vi "__Cloud List Menu Download Handler.vi"(7 "FileManager Data":T1, 8 "error in (no error)":errorcluster) -> (0 "error out":errorcluster)   [LabVIEW 2011]
doc: "Handles the download operation on the cloud list."
uses:
  __File manager Data type.ctl
  vi.lib/National Instruments/LabVIEW Interface for Amazon S3/LV Interface for Amazon S3.lvlib
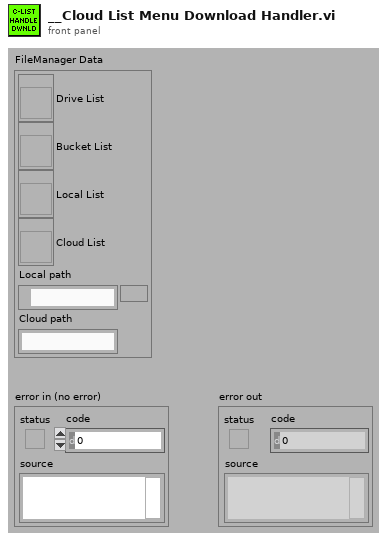
[diagram p1: front panel]
types:
  T1 = typedef "__File manager Data type.ctl" = cluster{"Drive List":refnum<vi>, "Bucket List":refnum<vi>, "Local List":refnum<vi>, "Cloud List":refnum<vi>, "Local path":path, "Cloud path":string}
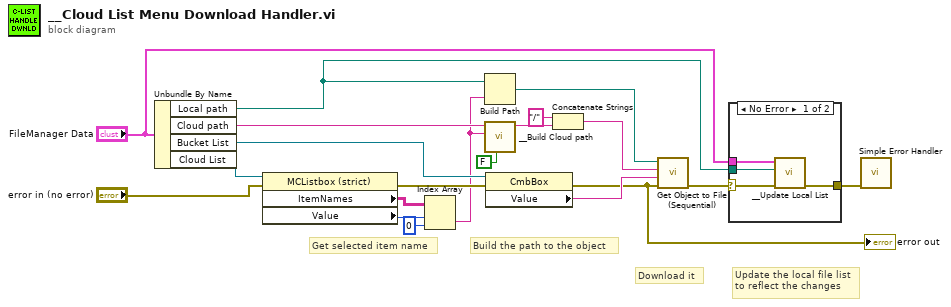
[diagram p0: block diagram]
diagram:
  # "Update the local file list\nto reflect the changes"
  # "Download it"
  # "Build the path to the object"
  # "Get selected item name"
  n1 = Unbundle By Name("FileManager Data") -> ("Local path"=w4:path, "Cloud path"=w13:string, "Bucket List"=w16:refnum<vi>, "Cloud List"=w20:refnum<vi>)
  n2 = property class="MCListbox (strict)"(reference=w20, error in="error in (no error)") -> (error out=w15:errorcluster, "ItemNames"=w19:string[][], "Value"=w18:i32)  [unwired: 1 out]
  n3 = Index Array(array=w19, index (row)=w18, index (col)=0 ("disabled index (col)")) -> (element=w10:string)
  n4 = Build Path(base path=w4, name or relative path=w10) -> (appended path=w7:path)
  n5 = call "__Build Cloud path.vi"("Folder?"=FALSE, "New Path element"=w10, "Current Cloud path"=w13) -> ("New Cloud path"=w11:string)  [unwired: 8 in]
  n6 = property class="CmbBox"(reference=w16, error in=w15) -> (error out=w2:errorcluster, "Value"=w9:string)  [unwired: 1 out]
  "error out" <- w2
  n7 = Concatenate Strings("/" ("string"), w11) -> (w8:string)
  n8 = call "Get Object to File (Sequential).vi"("error in (no error)"=w2, "Bucket"=w9, "Object Path"=w8, "File path"=w7) -> ("error out"=w6:errorcluster)  [unwired: 7 in]
  n9 = case shown="No Error" w6 {
    selector: w6 -> [w24 w25]
    tunnel: "FileManager Data" -> [w22 _]
    tunnel: w4 -> [w23 _]
    tunnel: [w21 w25] -> w3
    frame No Error {
      n10 = call "__Update Local List.vi"("error in (no error)"=w24, "Path to list"=w23, "FileManager Ctl Refs in"=w22) -> ("error out"=w21:errorcluster)  [unwired: 7 in, 1 out]
    }
    frame Error {
    }
  }
  n11 = call <vilib>:"Simple Error Handler.vi"("error in (no error)"=w3) -> ()  [unwired: 4 in, 5 out]
